vi "VI.set_control_lua.vi"(5 "LuaVIEW reference":T1) -> (15 "error out":errorcluster)   [LabVIEW 2012]
doc: "Sets the value of a control or indicator. No \"value changed\" event will be generated. Any data type that can be passed as compound data or occur as an element of compound data is supported.\nParameters:\nobj:self, VI object.\nstr:label, label of control/indicator to set.\nany:value, new value for control/indicator.\nErrors:\nNot a VI object.\nDead VI object.\nNo such control or indicator.\nData type of value does not match data type of control/indicator.\nData type of control/indicator not supported."
uses:
  typedefs/t_LuaVIEW Reference.ctl
  subvis/private/LuaVIEW Pull (object).vi
  subvis/private/LuaVIEW Pull (string).vi
  subvis/private/LuaVIEW Pull (flat data).vi
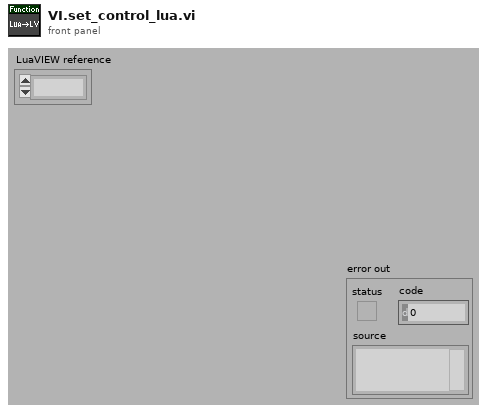
[diagram p1: front panel]
types:
  T1 = typedef "t_LuaVIEW Reference.ctl" = refnum<k1>
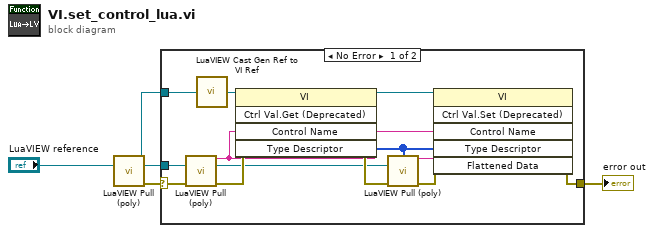
[diagram p0: block diagram]
diagram:
  n1 = call-poly "LuaVIEW Pull (poly).vi"("LuaVIEW reference in"="LuaVIEW reference") -> ("object refnum"=w3:refnum<vi>, "LuaVIEW reference out"=w1:T1, "error out"=w2:errorcluster)  [unwired: 11 in, 1 out]
  n2 = case shown="No Error" w2 {
    selector: w2 -> [w17 w19]
    tunnel: [w7 w19] -> w4
    tunnel: w3 -> [w18 _]
    tunnel: w1 -> [w16 _]
    frame No Error {
      n3 = call-poly "LuaVIEW Pull (poly).vi"("LuaVIEW reference in"=w16, "error in (no error)"=w17) -> ("string"=w6:string, "LuaVIEW reference out"=w8:T1, "error out"=w14:errorcluster)  [unwired: 11 in]
      n4 = call "LuaVIEW Cast Gen Ref to VI Ref.vi"("refnum in"=w18) -> ("refnum out"=w15:refnum<vi>)  [unwired: 14 in]
      n5 = invoke class="VI" method="Ctrl Val.Get (Deprecated)"(reference=w15, error in=w14, "Control Name"=w6) -> (reference out=w9:refnum<vi>, error out=w13:errorcluster, "Type Descriptor"=w12:i16[])  [unwired: 2 in, 2 out]
      n6 = call-poly "LuaVIEW Pull (poly).vi"("type descriptor"=w12, "LuaVIEW reference in"=w8, "error in (no error)"=w13) -> ("flat data"=w11:string, "error out"=w10:errorcluster)  [unwired: 10 in, 1 out]
      n7 = invoke class="VI" method="Ctrl Val.Set (Deprecated)"(reference=w9, error in=w10, "Control Name"=w6, "Type Descriptor"=w12, "Flattened Data"=w11) -> (error out=w7:errorcluster)  [unwired: 1 in, 5 out]
    }
    frame Error {
    }
  }
  "error out" <- w4
